vi "Exp Average.vi"(0 "s[i -1]":dbl, 2 "alfa":dbl, 5 "x":dbl) -> (4 "s[i]":dbl)   [LabVIEW 2019, in "AI.lvclass"]
uses:
  AI.lvclass
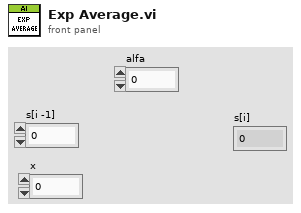
[diagram p1: front panel]
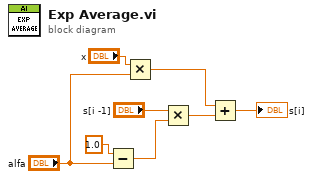
[diagram p0: block diagram]
diagram:
  n1 = Subtract(x=1.0, y="alfa") -> (x-y=w6:dbl)
  n2 = Multiply(x="x", y="alfa") -> (x*y=w7:dbl)
  n3 = Multiply(x="s[i -1]", y=w6) -> (x*y=w8:dbl)
  n4 = Add(x=w7, y=w8) -> (x+y=→"s[i]":dbl)
